vi "init.vi"(8 "error in":errorcluster, 10 "TBM module configuration in":refnum<class "TBM module configuration.lvclass">, 11 "tag bus configurable plugin module in":refnum<class "user tag bus module.lvclass">) -> (0 "error out":errorcluster, 1 "data allocations":T1, 2 "execution settings":T4, 3 "tag bus configurable plugin module out":refnum<class "user tag bus module.lvclass">)   [LabVIEW 2013, in "user tag bus module.lvclass"]
doc: "Provides an interface for initializing a module at runtime. While this interface performs no operations, a child should provide an override which may open any necessary references or sessions, allocate necessary memory, and perform any final configuration validataion before providing the full configuration <b>execution data</b> to the calling process."
uses:
  user tag bus module.lvclass
  <vilib>/NI/Tag Bus Module Framework/module configuration/TBM module configuration.lvclass
  <vilib>/NI/Tag Bus Module Framework/runtime/execution settings.ctl
  <vilib>/NI/Tag Bus Module Framework/channel/data tables.ctl
  <vilib>/NI/Tag Bus/dictionary/data dictionary.lvclass
  <vilib>/NI/Tag Bus/dictionary table pair.ctl
  <vilib>/NI/Tag Bus/table/data table.ctl
  configuration/user tag bus module configuration.lvclass
  state control.ctl
  configuration/user tag bus module configuration.lvclass/user tag bus module configuration.ctl
  <vilib>/NI/Tag Bus/tag/tag descriptor.lvclass/tag descriptor.ctl
  user tag bus module.lvclass/user tag bus module.ctl
  configuration/Read state module configuration.vi
  <vilib>/NI/Tag Bus/tag/read tag name.vi
  <vilib>/NI/Tag Bus/tag/read data type.vi
  <vilib>/NI/Tag Bus/dictionary/locate tag.vi
  <vilib>/NI/Tag Bus Module Framework/channel/TBM channel.lvclass
  <vilib>/NI/Tag Bus Module Framework/runtime/TBM module execution interface.lvclass
  <vilib>/NI/Tag Bus/tag bus.lvlib
  <vilib>/NI/Tag Bus/table/data table.lvlib
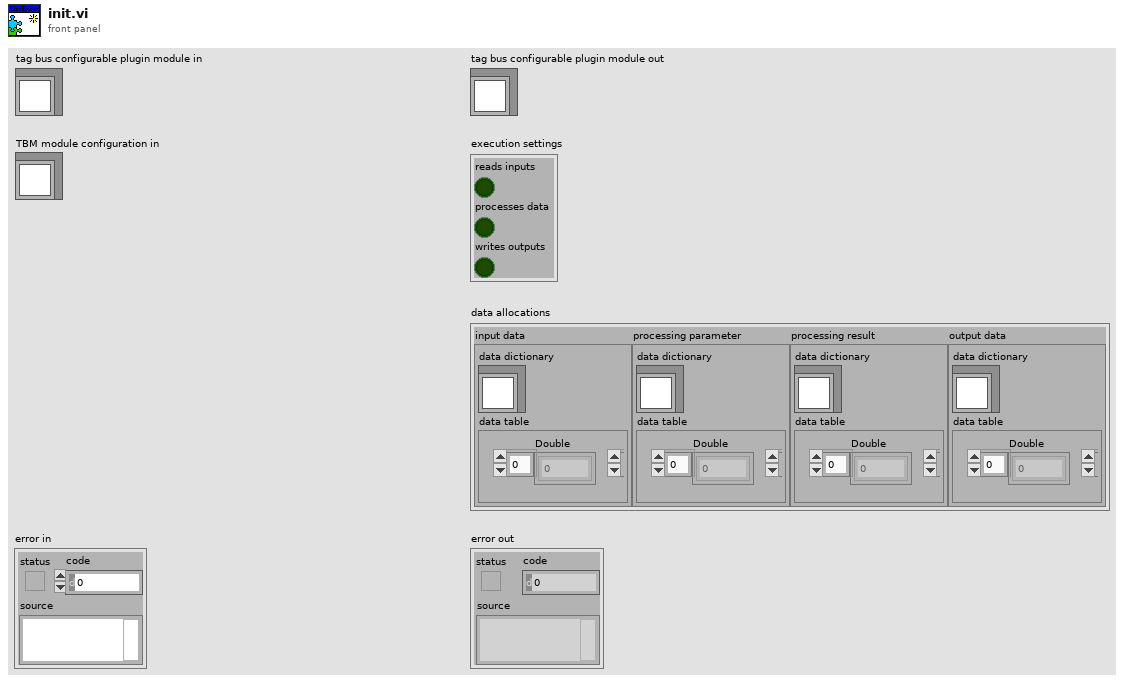
[diagram p1: front panel]
types:
  T1 = typedef "TBM channel.lvclass/data tables.ctl" = cluster{"input data":T2, "processing parameter":T2, "processing result":T2, "output data":T2}
  T2 = typedef "tag bus.lvlib/dictionary table pair.ctl" = cluster{"data dictionary":refnum<class "data dictionary.lvclass">, "data table":T3}
  T3 = typedef "tag bus.lvlib/data table.lvlib/data table.ctl" = cluster{"Double":dbl[], "Single":sgl[], "I64":i64[], "I32":i32[], "I16":i16[], "I8":i8[], "U64":u64[], "U32":u32[], "U16":u16[], "U8":u8[], "Boolean":bool[], "String":string[], "Array of Double":cluster{"DBL Array":dbl[]}[], "Array of Single":cluster{"SGL Array":sgl[]}[], "Array of I64":cluster{"I64 Array":i64[]}[], "Array of I32":cluster{"I32 Array":i32[]}[], "Array of I16":cluster{"I16 Array":i16[]}[], "Array of I8":cluster{"I8 Array":i8[]}[], "Array of U64":cluster{"U64 Array":u64[]}[], "Array of U32":cluster{"U32 Array":u32[]}[], "Array of U16":cluster{"U16 Array":u16[]}[], "Array of U8":cluster{"U8 Array":u8[]}[], "Array of Boolean":cluster{"Boolean Array":bool[]}[], "Array of String":cluster{"String Array":string[]}[]}
  T4 = typedef "TBM module execution interface.lvclass/execution settings.ctl" = cluster{"reads inputs":bool, "processes data":bool, "writes outputs":bool}
  T5 = typedef "user tag bus module.lvclass/state control.ctl" = cluster{"control index (dbl)":i32, "output index (dbl)":i32}
  T6 = typedef "user tag bus module configuration.lvclass/state module configuration.ctl" = cluster{"fixed input":refnum<class "TBM channel.lvclass">, "fixed output":refnum<class "TBM channel.lvclass">, "initial state":u8}
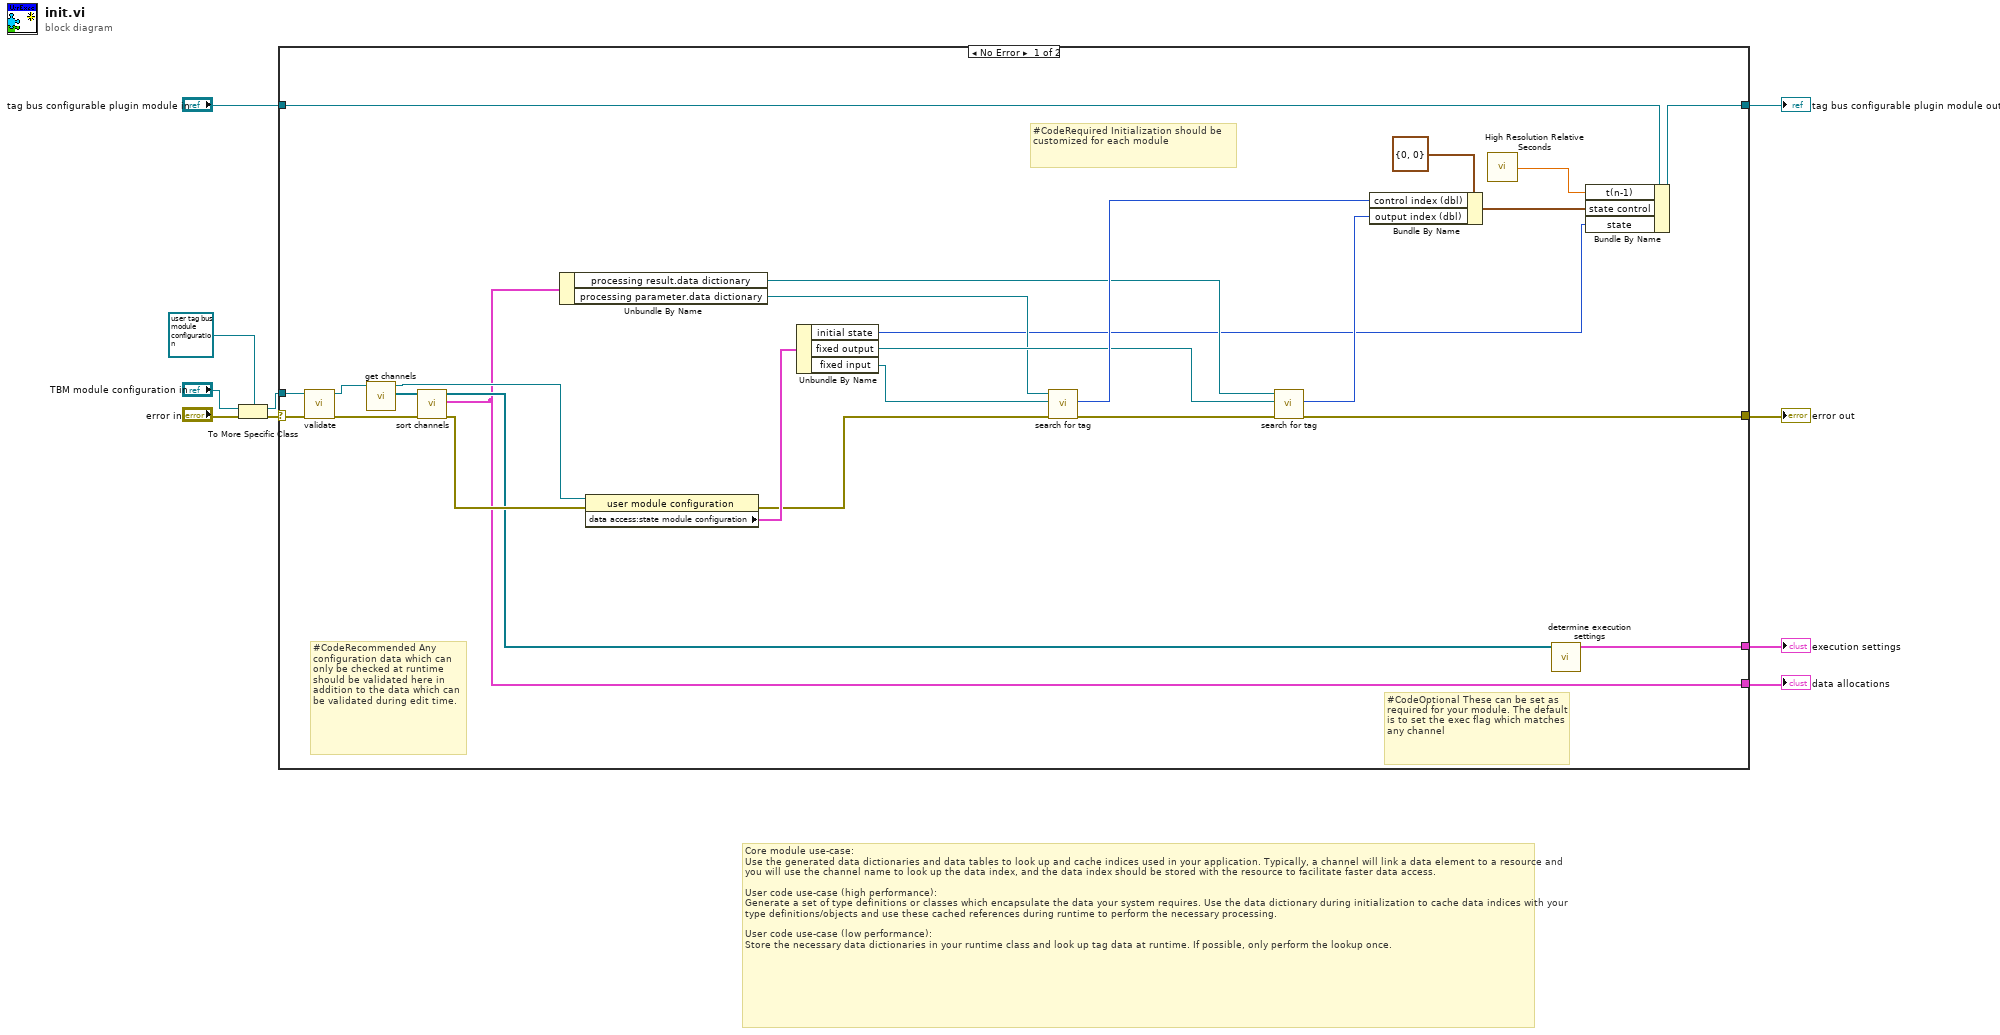
[diagram p0: block diagram]
diagram:
  # "Core module use-case:\nUse the generated data dictionaries and data tables to look up and cache indices used in your application. Typically, a channel will link a data element to a resource and you will use the channel name to look up the data index, and the data index should be stored with the resource to facilitate faster data access.\n\nUser code use-case (high performance):\nGenerate a set of type definitions or classes which encapsulate the data your system requires. Use the data dictionary during initialization to cache data indices with your type definitions/objects and use these cached references during runtime to perform the necessary processing.\n\nUser code use-case (low performance):\nStore the necessary data dictionaries in your runtime class and look up tag data at runtime. If possible, only perform the lookup once."
  n1 = To More Specific Class(target class=refnum<class "user tag bus module configuration.lvclass"> refnum ("Synchronous module configuration"), reference="TBM module configuration in", error in="error in") -> (specific class reference=w9:refnum<class "user tag bus module configuration.lvclass">, error out=w10:errorcluster)
  n2 = case shown="No Error" w10 {
    selector: w10 -> [w31 w37]
    tunnel: w9 -> [w30 _]
    tunnel: "tag bus configurable plugin module in" -> [w36 w38]
    tunnel: [w25 w38] -> w4
    tunnel: [w17 w37] -> w3
    tunnel: [w26 _] -> w1
    tunnel: [w34 _] -> w2
    frame No Error {
      # "#CodeRecommended Any configuration data which can only be checked at runtime should be validated here in addition to the data which can be validated during edit time."
      # "#CodeOptional These can be set as required for your module. The default is to set the exec flag which matches any channel"
      # "#CodeRequired Initialization should be customized for each module"
      n3 = call-dynamic "validate.vi"("error in"=w31, "tag bus configurable plugin module configuration in"=w30) -> ("error out"=w32:errorcluster, "tag bus configurable plugin module configuration out"=w29:refnum<class "user tag bus module configuration.lvclass">)  [unwired: 8 in]
      n4 = call-dynamic "get channels.vi"("user tag bus module configuration In"=w29) -> ("channels"=w28:refnum<class "TBM channel.lvclass">[], "user tag bus module configuration Out"=w27:refnum<class "user tag bus module configuration.lvclass">)  [unwired: 9 in]
      n5 = call <vilib>:"sort channels.vi"("error in"=w32, "channels in"=w28) -> ("error out"=w35:errorcluster, "data allocations"=w26:T1, "channels out"=w33:refnum<class "TBM channel.lvclass">[])  [unwired: 7 in]
      n6 = Unbundle By Name(w26) -> ("processing result.data dictionary"=w18:refnum<class "data dictionary.lvclass">, "processing parameter.data dictionary"=w13:refnum<class "data dictionary.lvclass">)
      n7 = property class="user module configuration"(reference=w27, error in=w35) -> (error out=w14:errorcluster, "data access:state module configuration"=w24:T6)  [unwired: 1 out]
      n8 = Unbundle By Name(w24) -> ("initial state"=w11:u8, "fixed output"=w19:refnum<class "TBM channel.lvclass">, "fixed input"=w12:refnum<class "TBM channel.lvclass">)
      n9 = call <vilib>:"search for tag.vi"("error in"=w14, "system tag"=w12, "data dictionary in"=w13) -> ("error out"=w15:errorcluster, "index"=w20:i32)  [unwired: 6 in, 1 out]
      n10 = call <vilib>:"search for tag.vi"("error in"=w15, "system tag"=w19, "data dictionary in"=w18) -> ("error out"=w17:errorcluster, "index"=w21:i32)  [unwired: 6 in, 1 out]
      n11 = Bundle By Name(cluster=T5 {"control index (dbl)"=0, "output index (dbl)"=0} ("state control"), "control index (dbl)"=w20, "output index (dbl)"=w21) -> (w22:T5)
      n12 = call <vilib>:"High Resolution Relative Seconds.vi"() -> ("relative seconds"=w16:dbl)
      n13 = call <vilib>:"determine execution settings.vi"("channels"=w33) -> ("execution settings"=w34:T4)  [unwired: 10 in]
      n14 = Bundle By Name(cluster=w36, "t(n-1)"=w16, "state control"=w22, "state"=w11) -> (w25:refnum<class "user tag bus module.lvclass">)
    }
    frame Error {
    }
  }
  "error out" <- w3
  "tag bus configurable plugin module out" <- w4
  "execution settings" <- w2
  "data allocations" <- w1
